vi "Chip Select.vi"(1 "Chip Select":T1=enum."None") -> ()   [LabVIEW 2018]
uses:
  Type Defs/Chip Select.ctl
  <vilib>/rvi/eio/common/nirviEmuTemplateMethod_errors.vi
  <vilib>/eio/EIONode/EIONode.xnode
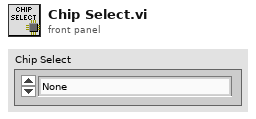
[diagram p1: front panel]
types:
  T1 = typedef "Chip Select.ctl" = enum16{"Axial Field", "None", "dsPIC Corona"}
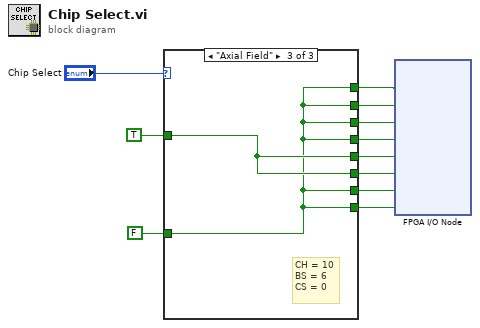
[diagram p0: block diagram]
diagram:
  n1 = case shown="\"Axial Field\"" "Chip Select" {
    tunnel: TRUE -> [w13 w14 w17]
    tunnel: FALSE -> [w12 w15 w16]
    tunnel: [w13 w14 w16] -> w8
    tunnel: [w13 w15 w16] -> w7
    tunnel: [w13 w15 w16] -> w6
    tunnel: [w12 w15 w16] -> w5
    tunnel: [w12 w15 w17] -> w4
    tunnel: [w12 w14 w17] -> w3
    tunnel: [w12 w14 w16] -> w2
    tunnel: [w12 w15 w16] -> w1
    frame "None", Default {
    }
    frame "dsPIC Corona" {
      # "Board = 12\nCS = 0"
    }
    frame "Axial Field" {
      # "CH = 10\nBS = 6\nCS = 0"
    }
  }
  n2 = xnode "FPGA I/O Node"("CS0"=w8, "CS1"=w7, "CS2"=w6, "BS0"=w5, "BS1"=w4, "BS2"=w3, "BS3"=w2, "BS4"=w1) -> ()  [unwired: 8 in, 8 out]
